vi "MoveMultipleJogSteps.vi"(8 "error in (no error)":errorcluster, 9 "Step Amounts":dbl, 10 "direction":i32(ring)=1 items=["Forward"=1, "Backward"=2], 11 "ThorlabsLabJack in":refnum<class "ThorlabsLabJack.lvclass">) -> (0 "error out":errorcluster, 3 "ThorlabsLabJack out":refnum<class "ThorlabsLabJack.lvclass">)   [LabVIEW 2018, in "ThorlabsLabJack.lvlib" / "ThorlabsLabJack.lvclass"]
uses:
  ThorlabsLabJack.lvclass
  ThorlabsLabJack.lvclass/ThorlabsLabJack.ctl
  C:/Projects/LabVIEW/In-Progress/Chetan Malpure/Axis/Thorlabs LabJack/Drivers/Thorlabs.MotionControl.IntegratedStepperMotorsCLI.dll
  Drivers/Thorlabs.MotionControl.IntegratedStepperMotorsCLI.dll
  674df32a-57a9-47a4-a3c5-78e16ca3a594.vi
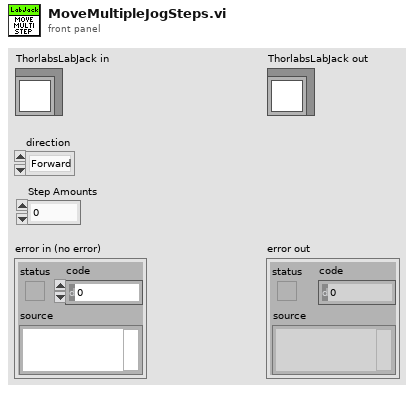
[diagram p1: front panel]
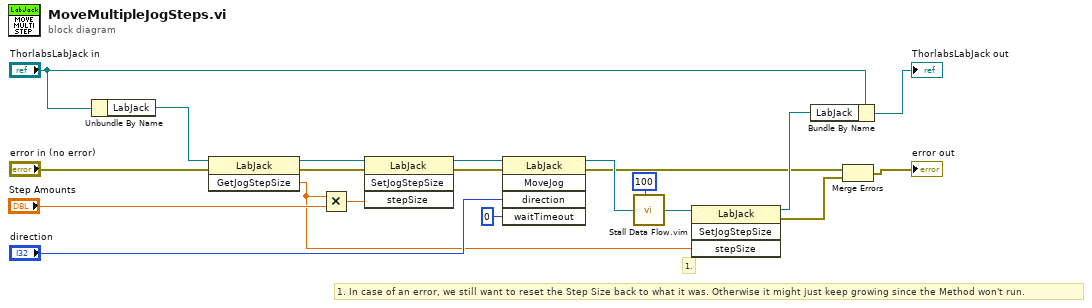
[diagram p0: block diagram]
diagram:
  # "1."
  # "1. In case of an error, we still want to reset the Step Size back to what it was. Otherwise it might just keep growing since the Method won't run."
  n1 = Unbundle By Name("ThorlabsLabJack in") -> ("LabJack"=w17:refnum<k24>)
  n2 = invoke class="LabJack" method="GetJogStepSize"(reference=w17, error in="error in (no error)") -> (reference out=w14:refnum<k24>, error out=w13:errorcluster, "GetJogStepSize"=w1:dbl)  [unwired: 1 in]
  n3 = Multiply(x=w1, y="Step Amounts") -> (x*y=w12:dbl)
  n4 = invoke class="LabJack" method="SetJogStepSize"(reference=w14, error in=w13, "stepSize"=w12) -> (reference out=w11:refnum<k24>, error out=w10:errorcluster)  [unwired: 1 in, 2 out]
  n5 = invoke class="LabJack" method="MoveJog"(reference=w11, error in=w10, "direction"="direction", "waitTimeout"=0) -> (reference out=w7:refnum<k24>, error out=w2:errorcluster)  [unwired: 1 in, 3 out]
  n6 = call "Stall Data Flow.vim"("value in"=w7, "milliseconds to wait"=u32 100) -> ("value out"=w6:refnum<k24>)  [unwired: 1 out]
  n7 = invoke class="LabJack" method="SetJogStepSize"(reference=w6, "stepSize"=w1) -> (reference out=w5:refnum<k24>, error out=w4:errorcluster)  [unwired: 2 in, 2 out]
  n8 = Bundle By Name(cluster="ThorlabsLabJack in", "LabJack"=w5) -> (→"ThorlabsLabJack out":refnum<class "ThorlabsLabJack.lvclass">)
  n9 = Merge Errors(w2, w4) -> (→"error out":errorcluster)
